vi "LCR_Logfile.vi"(4 "Secondary Measurement":dbl, 6 "Primary Measurement":dbl, 7 "Time Stamp":timestamp format="%<%x %.3X>T", 8 "error in":errorcluster, 9 "FilePrefix":string, 10 "Config_In":T1={"General"={"Config.ini"=path "", "Default Logging Path"=path ""}, "Hardware"={"LCR VISA COM"="", "Measure Rate (1/s)"=0, "Reset on Load?"=FALSE, "Measure Profile"=path ""}, "HM8118 Current Profile"={"Bias Profile"={" Bias Source (OFF)"=0, " Bias Type (Voltage)"=0, "Bias Level (0)"=0.0}, "Measurement Profile"={"Operation Mode (0: Auto)"=0, "Circuit Type (2: Auto)"=2, "Manual Range (1:Range 1 and 25 Ohms)"=1, "Auto Range (T: Enable)"=TRUE}, "Signal Profile"={"Frequency (1kHz)"=1000.0, "Measuring Voltage (1V)"=1.0}, "Integration Profile"={"Averaging (0: Off)"=0, "Averaging Number (2)"=2, "Time (100ms)"=100, "Rate (0: Fast)"=0}, "Trigger Profile"={"Trigger Mode (0: Continuous)"=0}}, "HM8118 New Profile"={"Bias Profile"={" Bias Source (OFF)"=0, " Bias Type (Voltage)"=0, "Bias Level (0)"=0.0}, "Measurement Profile"={"Operation Mode (0: Auto)"=0, "Circuit Type (2: Auto)"=2, "Manual Range (1:Range 1 and 25 Ohms)"=1, "Auto Range (T: Enable)"=TRUE}, "Signal Profile"={"Frequency (1kHz)"=1000.0, "Measuring Voltage (1V)"=1.0}, "Integration Profile"={"Averaging (0: Off)"=0, "Averaging Number (2)"=2, "Time (100ms)"=100, "Rate (0: Fast)"=0}, "Trigger Profile"={"Trigger Mode (0: Continuous)"=0}}, "Operation"={"Operation Mode"=enum."Logging"}} {"HM8118 New Profile"."Trigger Profile"."Trigger Mode (0: Continuous)" items=["Continuous", "Manual", "External"]; "HM8118 New Profile"."Integration Profile"."Rate (0: Fast)" items=["Fast", "Medium", "Slow"]; "HM8118 New Profile"."Integration Profile"."Time (100ms)" min=1 max=999; "HM8118 New Profile"."Integration Profile"."Averaging Number (2)" min=2 max=99; "HM8118 New Profile"."Integration Profile"."Averaging (0: Off)" items=["Off", "Normal", "Averaging"]; "HM8118 New Profile"."Signal Profile"."Measuring Voltage (1V)" min=0.05 max=1.5 step=0.01; "HM8118 New Profile"."Signal Profile"."Frequency (1kHz)" min=20.0 max=200000.0; "HM8118 New Profile"."Measurement Profile"."Manual Range (1:Range 1 and 25 Ohms)" items=["Range 1 and 25 Ohms"=1, "Range 2 and 25 Ohms"=2, "Range 3 and 400 Ohms"=3, "Range 4 and 6.4 kOhms"=4, "Range 5 and 100kOhms"=5, "Range 6 and 100kOhms"=6]; "HM8118 New Profile"."Measurement Profile"."Circuit Type (2: Auto)" items=["Series", "Parallel", "Auto"]; "HM8118 New Profile"."Measurement Profile"."Operation Mode (0: Auto)" items=["Auto", "L+Q", "L+R", "C+D", "C+R", "R+Q", "Z+Theta", "Y+Theta", "R+X", "G+B", "N+Theta", "M"]; "HM8118 New Profile"."Bias Profile"."Bias Type (Voltage)" items=["Voltage", "Current"]; "HM8118 New Profile"."Bias Profile"."Bias Source (OFF)" items=["Off", "Internal", "External"]; "HM8118 Current Profile"."Trigger Profile"."Trigger Mode (0: Continuous)" items=["Continuous", "Manual", "External"]; "HM8118 Current Profile"."Integration Profile"."Rate (0: Fast)" items=["Fast", "Medium", "Slow"]; "HM8118 Current Profile"."Integration Profile"."Time (100ms)" min=1 max=999; "HM8118 Current Profile"."Integration Profile"."Averaging Number (2)" min=2 max=99; "HM8118 Current Profile"."Integration Profile"."Averaging (0: Off)" items=["Off", "Normal", "Averaging"]; "HM8118 Current Profile"."Signal Profile"."Measuring Voltage (1V)" min=0.05 max=1.5 step=0.01; "HM8118 Current Profile"."Signal Profile"."Frequency (1kHz)" min=20.0 max=200000.0; "HM8118 Current Profile"."Measurement Profile"."Manual Range (1:Range 1 and 25 Ohms)" items=["Range 1 and 25 Ohms"=1, "Range 2 and 25 Ohms"=2, "Range 3 and 400 Ohms"=3, "Range 4 and 6.4 kOhms"=4, "Range 5 and 100kOhms"=5, "Range 6 and 100kOhms"=6]; "HM8118 Current Profile"."Measurement Profile"."Circuit Type (2: Auto)" items=["Series", "Parallel", "Auto"]; "HM8118 Current Profile"."Measurement Profile"."Operation Mode (0: Auto)" items=["Auto", "L+Q", "L+R", "C+D", "C+R", "R+Q", "Z+Theta", "Y+Theta", "R+X", "G+B", "N+Theta", "M"]; "HM8118 Current Profile"."Bias Profile"."Bias Type (Voltage)" items=["Voltage", "Current"]; "HM8118 Current Profile"."Bias Profile"."Bias Source (OFF)" items=["Off", "Internal", "External"]}) -> (0 "error out":errorcluster, 2 "Config_Out":T1={"General"={"Config.ini"=path "", "Default Logging Path"=path ""}, "Hardware"={"LCR VISA COM"="", "Measure Rate (1/s)"=0, "Reset on Load?"=FALSE, "Measure Profile"=path ""}, "HM8118 Current Profile"={"Bias Profile"={" Bias Source (OFF)"=0, " Bias Type (Voltage)"=0, "Bias Level (0)"=0.0}, "Measurement Profile"={"Operation Mode (0: Auto)"=0, "Circuit Type (2: Auto)"=2, "Manual Range (1:Range 1 and 25 Ohms)"=1, "Auto Range (T: Enable)"=TRUE}, "Signal Profile"={"Frequency (1kHz)"=1000.0, "Measuring Voltage (1V)"=1.0}, "Integration Profile"={"Averaging (0: Off)"=0, "Averaging Number (2)"=2, "Time (100ms)"=100, "Rate (0: Fast)"=0}, "Trigger Profile"={"Trigger Mode (0: Continuous)"=0}}, "HM8118 New Profile"={"Bias Profile"={" Bias Source (OFF)"=0, " Bias Type (Voltage)"=0, "Bias Level (0)"=0.0}, "Measurement Profile"={"Operation Mode (0: Auto)"=0, "Circuit Type (2: Auto)"=2, "Manual Range (1:Range 1 and 25 Ohms)"=1, "Auto Range (T: Enable)"=TRUE}, "Signal Profile"={"Frequency (1kHz)"=1000.0, "Measuring Voltage (1V)"=1.0}, "Integration Profile"={"Averaging (0: Off)"=0, "Averaging Number (2)"=2, "Time (100ms)"=100, "Rate (0: Fast)"=0}, "Trigger Profile"={"Trigger Mode (0: Continuous)"=0}}, "Operation"={"Operation Mode"=enum."Logging"}} {"HM8118 New Profile"."Trigger Profile"."Trigger Mode (0: Continuous)" items=["Continuous", "Manual", "External"]; "HM8118 New Profile"."Integration Profile"."Rate (0: Fast)" items=["Fast", "Medium", "Slow"]; "HM8118 New Profile"."Integration Profile"."Time (100ms)" min=1 max=999; "HM8118 New Profile"."Integration Profile"."Averaging Number (2)" min=2 max=99; "HM8118 New Profile"."Integration Profile"."Averaging (0: Off)" items=["Off", "Normal", "Averaging"]; "HM8118 New Profile"."Signal Profile"."Measuring Voltage (1V)" min=0.05 max=1.5 step=0.01; "HM8118 New Profile"."Signal Profile"."Frequency (1kHz)" min=20.0 max=200000.0; "HM8118 New Profile"."Measurement Profile"."Manual Range (1:Range 1 and 25 Ohms)" items=["Range 1 and 25 Ohms"=1, "Range 2 and 25 Ohms"=2, "Range 3 and 400 Ohms"=3, "Range 4 and 6.4 kOhms"=4, "Range 5 and 100kOhms"=5, "Range 6 and 100kOhms"=6]; "HM8118 New Profile"."Measurement Profile"."Circuit Type (2: Auto)" items=["Series", "Parallel", "Auto"]; "HM8118 New Profile"."Measurement Profile"."Operation Mode (0: Auto)" items=["Auto", "L+Q", "L+R", "C+D", "C+R", "R+Q", "Z+Theta", "Y+Theta", "R+X", "G+B", "N+Theta", "M"]; "HM8118 New Profile"."Bias Profile"."Bias Type (Voltage)" items=["Voltage", "Current"]; "HM8118 New Profile"."Bias Profile"."Bias Source (OFF)" items=["Off", "Internal", "External"]; "HM8118 Current Profile"."Trigger Profile"."Trigger Mode (0: Continuous)" items=["Continuous", "Manual", "External"]; "HM8118 Current Profile"."Integration Profile"."Rate (0: Fast)" items=["Fast", "Medium", "Slow"]; "HM8118 Current Profile"."Integration Profile"."Time (100ms)" min=1 max=999; "HM8118 Current Profile"."Integration Profile"."Averaging Number (2)" min=2 max=99; "HM8118 Current Profile"."Integration Profile"."Averaging (0: Off)" items=["Off", "Normal", "Averaging"]; "HM8118 Current Profile"."Signal Profile"."Measuring Voltage (1V)" min=0.05 max=1.5 step=0.01; "HM8118 Current Profile"."Signal Profile"."Frequency (1kHz)" min=20.0 max=200000.0; "HM8118 Current Profile"."Measurement Profile"."Manual Range (1:Range 1 and 25 Ohms)" items=["Range 1 and 25 Ohms"=1, "Range 2 and 25 Ohms"=2, "Range 3 and 400 Ohms"=3, "Range 4 and 6.4 kOhms"=4, "Range 5 and 100kOhms"=5, "Range 6 and 100kOhms"=6]; "HM8118 Current Profile"."Measurement Profile"."Circuit Type (2: Auto)" items=["Series", "Parallel", "Auto"]; "HM8118 Current Profile"."Measurement Profile"."Operation Mode (0: Auto)" items=["Auto", "L+Q", "L+R", "C+D", "C+R", "R+Q", "Z+Theta", "Y+Theta", "R+X", "G+B", "N+Theta", "M"]; "HM8118 Current Profile"."Bias Profile"."Bias Type (Voltage)" items=["Voltage", "Current"]; "HM8118 Current Profile"."Bias Profile"."Bias Source (OFF)" items=["Off", "Internal", "External"]})   [LabVIEW 2021]
uses:
  Config_Cluster.ctl
  Mode_Enum.ctl
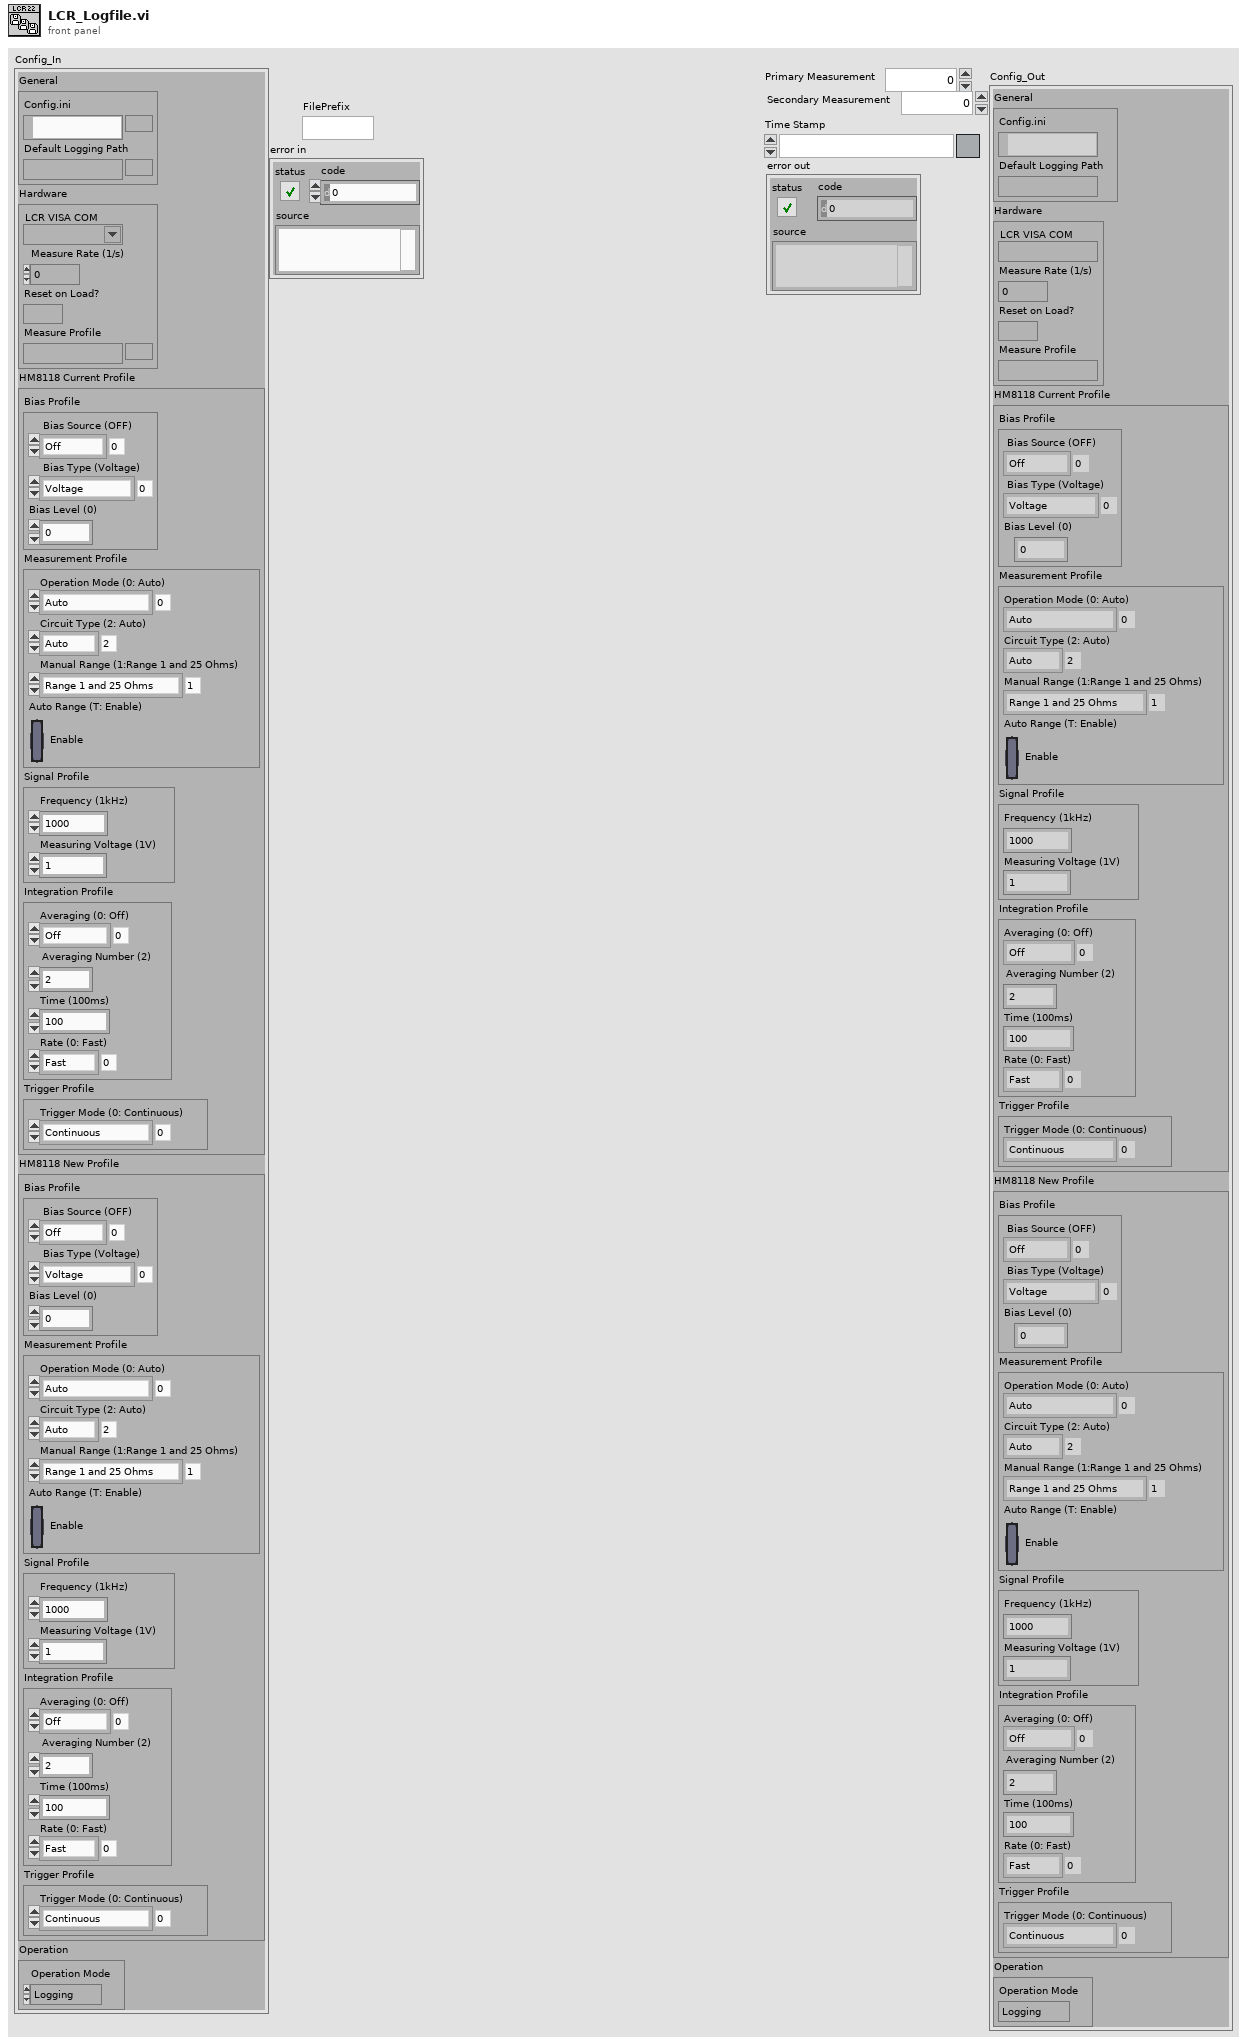
[diagram p1: front panel]
types:
  T1 = typedef "Config_Cluster.ctl" = cluster{"General":cluster{"Config.ini":path, "Default Logging Path":path}, "Hardware":cluster{"LCR VISA COM":refnum<visa-resource-name>, "Measure Rate (1/s)":i32, "Reset on Load?":bool, "Measure Profile":path}, "HM8118 Current Profile":cluster{"Bias Profile":cluster{" Bias Source (OFF)":u8, " Bias Type (Voltage)":u8, "Bias Level (0)":dbl}, "Measurement Profile":cluster{"Operation Mode (0: Auto)":u16, "Circuit Type (2: Auto)":u16, "Manual Range (1:Range 1 and 25 Ohms)":u8, "Auto Range (T: Enable)":bool}, "Signal Profile":cluster{"Frequency (1kHz)":dbl, "Measuring Voltage (1V)":dbl}, "Integration Profile":cluster{"Averaging (0: Off)":u16, "Averaging Number (2)":i32, "Time (100ms)":i32, "Rate (0: Fast)":u16}, "Trigger Profile":cluster{"Trigger Mode (0: Continuous)":u16}}, "HM8118 New Profile":cluster{"Bias Profile":cluster{" Bias Source (OFF)":u8, " Bias Type (Voltage)":u8, "Bias Level (0)":dbl}, "Measurement Profile":cluster{"Operation Mode (0: Auto)":u16, "Circuit Type (2: Auto)":u16, "Manual Range (1:Range 1 and 25 Ohms)":u8, "Auto Range (T: Enable)":bool}, "Signal Profile":cluster{"Frequency (1kHz)":dbl, "Measuring Voltage (1V)":dbl}, "Integration Profile":cluster{"Averaging (0: Off)":u16, "Averaging Number (2)":i32, "Time (100ms)":i32, "Rate (0: Fast)":u16}, "Trigger Profile":cluster{"Trigger Mode (0: Continuous)":u16}}, "Operation":cluster{"Operation Mode":T2}}
  T2 = typedef "Mode_Enum.ctl" = enum16{"Logging", "Idle-Off", "Idle"}
  T3 = enum16{"open", "replace", "create", "open or create", "replace or create", "replace or create with confirmation"}
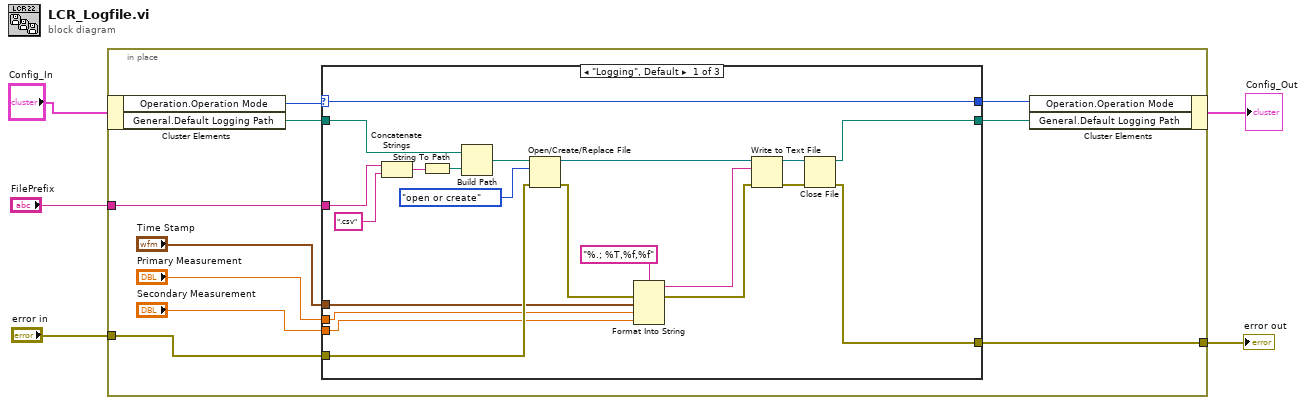
[diagram p0: block diagram]
diagram:
  n1 = in-place {
    in-place-border: "FilePrefix" -> [w12]
    in-place-border: "error in" -> [w11]
    in-place-border: [w6] -> w2
    n2 = in-place-cluster #1("Config_In") -> ("Operation.Operation Mode"=w15:T2, "General.Default Logging Path"=w13:path)
    n3 = case shown="\"Logging\", Default" w15 {
      selector: w15 -> [w36 w39 w42]
      tunnel: [w36 w39 w42] -> w14
      tunnel: w13 -> [w35 w38 w41]
      tunnel: w12 -> [w32 _ _]
      tunnel: w11 -> [w28 w37 w40]
      tunnel: "Time Stamp" -> [w23 _ _]
      tunnel: "Primary Measurement" -> [w22 _ _]
      tunnel: "Secondary Measurement" -> [w21 _ _]
      tunnel: [w17 w38 w41] -> w7
      tunnel: [w16 w37 w40] -> w6
      frame "Logging", Default {
        n4 = Concatenate Strings(w32, ".csv") -> (w31:string)
        n5 = String To Path(string=w31) -> (path=w34:path)
        n6 = Build Path(base path=w35, name or relative path=w34) -> (appended path=w30:path)
        n7 = Open/Create/Replace File(file path (use dialog)=w30, error in=w28, operation (0:open)=T3."open or create") -> (refnum out=w27:refnum<file>, error out=w25:errorcluster)  [unwired: 3 in, 1 out]
        n8 = Format Into String(format string="%.; %T,%f,%f", error in=w25, w23, w22, w21) -> (resulting string=w20:string, error out=w24:errorcluster)  [unwired: 1 in]
        n9 = Write to Text File(file (use dialog)=w27, text=w20, error in=w24) -> (refnum out=w18:refnum<file>, error out=w19:errorcluster)  [unwired: 1 in, 1 out]
        n10 = Close File(refnum=w18, error in=w19) -> (path=w17:path, error out=w16:errorcluster)
      }
      frame "Idle-Off" {
      }
      frame "Idle" {
      }
    }
    n11 = in-place-cluster #1("Operation.Operation Mode"=w14, "General.Default Logging Path"=w7) -> (→"Config_Out":T1)
  }
  "error out" <- w2
